vi "CH_LM Action Configuration Catalog.vi"(0 "Meter Index":i32, 5 "error in (no error)":errorcluster, 7 "Timeout / ms (3000)":i32=3000, 9 "Lock Timeout / ms (1000)":i32=1000) -> (11 "Lock timed out":bool, 14 "Meter Index":i32, 16 "Configuration Catalog":string[](array[string]), 19 "error out":errorcluster)   [LabVIEW 2012, in "CH_LM.lvlib"]
doc: "This query will get the list of stored configuration files that were saved by the user."
uses:
  CH_LM.lvlib
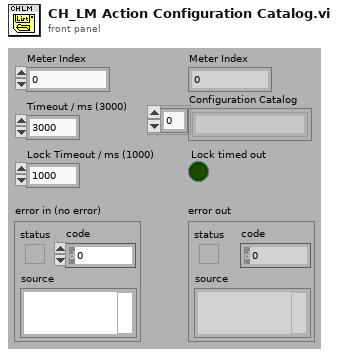
[diagram p1: front panel]
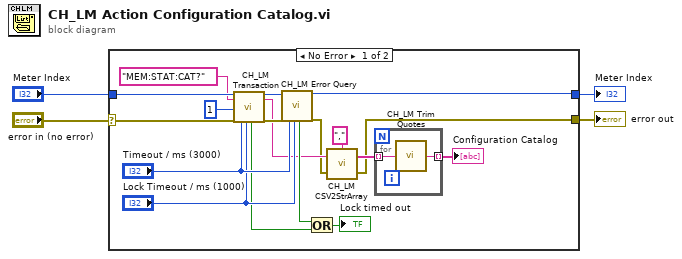
[diagram p0: block diagram]
diagram:
  n1 = case shown="No Error" "error in (no error)" {
    selector: "error in (no error)" -> [w22 w26]
    tunnel: [w6 w26] -> w4
    tunnel: "Meter Index" -> [w21 w25]
    tunnel: [w16 w25] -> w1
    frame No Error {
      n2 = call "CH_LM Transaction.vi"("Meter Index"=w21, "Command String"="MEM:STAT:CAT?", "NofStrings (-1:all)"=1, "error in (no error)"=w22, "Timeout / ms (3000)"="Timeout / ms (3000)", "Lock Timeout / ms (1000)"="Lock Timeout / ms (1000)") -> ("Lock timed out"=w12:bool, "Meter Index"=w17:i32, "Response"=w10:string, "error out"=w18:errorcluster)  [unwired: 10 out]
      n3 = call "CH_LM Error Query.vi"("Meter Index"=w17, "error in (no error)"=w18, "Timeout / ms (3000)"="Timeout / ms (3000)", "Lock Timeout / ms (1000)"="Lock Timeout / ms (1000)") -> ("Lock timed out"=w13:bool, "Meter Index"=w16:i32, "error out"=w7:errorcluster)  [unwired: 13 out]
      n4 = Or(x=w13, y=w12) -> (x .or. y?=→"Lock timed out":bool)
      n5 = call "CH_LM CSV2StrArray.vi"("error in (no error)"=w7, "CSL"=w10, "Separator (,)"=",") -> ("error out"=w6:errorcluster, "Strings"=w8:string[])
      n6 = for {
        tunnel: w8 -> [w24] mode=indexing
        tunnel: [w23] -> w5 mode=indexing
        n7 = call "CH_LM Trim Quotes.vi"("string"=w24) -> ("trimmed string"=w23:string)  [unwired: 1 in]
      }
      "Configuration Catalog" <- w5
    }
    frame Error {
    }
  }
  "error out" <- w4
  "Meter Index" <- w1
